vi "Window-Calibration toolbox.vi"() -> ()   [LabVIEW 2017]
uses:
  Configuration code/Calibration/ToolBox/TypeDefs/Current Calibration Parameters.ctl
  Configuration code/Calibration/ToolBox/TypeDefs/ProcedureState.ctl
  Typedefs/Objective selector control enum.ctl
  <vilib>/Math Plots/3D Math Plots/3D Surface/3D Surface XCtrl/3D Surface.xctl
  <vilib>/vision/Image Controls.llb/IMAQ Image.ctl
  Configuration code/Calibration/ToolBox/TypeDefs/Procedure_State.ctl
  Configuration code/Calibration/ToolBox/TypeDefs/Control Plane.ctl
  Typedefs/HW config states enum.ctl
  Peripherals Control/XYZ Stage/Typedefs/XYZ stage data.ctl
  Peripherals Control/XYZ Stage/Typedefs/XYZ stage states.ctl
  Peripherals Control/XYZ Stage/Typedefs/XYZ channel ring.ctl
  Global Variables/General Globals.vi
  Configuration code/Calibration/Globals/gl_Calibration globals.vi
  Global Variables/gl_UI Ctrl Refs.vi
  <vilib>/Math Plots/3D Math Plots/3D Surface/3D Surface Datatype/Public/Plot Helper (Matrix).vi
  <resource>/objmgr/IMAQImage.rc
  <vilib>/GPower/Array/GPArray.lvlib
  Global Variables/gl_Queues.vi
  <vilib>/Math Plots/3D Math Plots/3D Surface/3D Surface Datatype/3D Surface Datatype.lvclass
  <vilib>/GPower/Array/Library/Create/Random/CreateRandomI8.vi
panel:
  out "Focal Plane":sgl format="Z:%#_g"
  in  "Set focal plane":bool
  out "Z plane exec time":u32
  out "Stage XYZ Position":cluster{"X":sgl, "Y":sgl, "Z":sgl}
  out "3D Surface":refnum<class "3D Plot Datatype.lvclass">[](xcontrol)
  out "Intensity Graph":i16[][](graph)
  out "Image Pixels (I16)":i16[][](array[numeric])
  out "Stage Zeroed ? 2":bool
  out "AOL Z values":i32[](array[numeric])
  out "Motor Z values":i32[](array[numeric])
  out "mini steps":dbl=100.0
  out "LL":dbl=100.0 format="%#_g µm"
  out "UL":dbl=100.0 format="%#_g µm"
  in  "miniStep size":dbl=100.0 format="%#_g µm"
  in  "Sequence":bool
  out "Stage Zeroed ?":bool
  out "Z":sgl format="Z:%#_g"
  out "Y":sgl format="Y:%#_g"
  out "X":sgl format="X:%#_g"
  out "Progress":u8(slide) scale=0.0..21.0
  in  "Step Size":dbl=100.0 format="%#_g µm"
  in  "Natural Plane":bool
  in  "Move Down":bool
  in  "Move Up":bool
  in  "Current Objective":T1="Olympus  20X"
  out "error out":errorcluster
  out "Procedure":T2
  in  "Auto Focus":bool
  in  "Signal Channel":enum16{"Red", "Green"}(ring)
  in  "Message_FrontPanel":string
  in  "Cancel":bool
  in  "Abort":bool
  in  "Next":bool
  in  "N":i32=512
  in  "Reload":bool
  out "Stop_Ind":bool
  in  "Save config.ini":bool
  in  "Exit":bool
  in  "Calibration Tab":T3(tab)
  in  "Live Image intensity":cluster{i16, i16}(slide)={0, 2048} scale=0.0..4095.0
  in  "Visible(Grid)":bool
  in  "Grid Lines":u32=2 min=2 max=10 step=1
  out "Image":T4(plugin-control)
  out "Array":T4[](array[plugin-control])
  out "Analysis Graph":cluster{"X":dbl, "Y":dbl}[](graph)
  out "PSF Plot":cluster{"X":dbl, "Y":dbl}[](graph)
  out "PSF Image":T4(plugin-control)
  in  "Objectives":string(tree)
  out "Calibration.ini Path":path
  out "Calibration.ini":string
  in  "Step details":string
  in  "Step No":T5(ring)
  in  "Pockels Cell Value for pointing mode":dbl
  in  "auto-set pockel":bool
  in  "Calibration_min":dbl
  in  "Calibration_max":dbl
  in  "Search_min":dbl
  in  "Search_max":dbl
  in  "Testing Range (Norm)_max":dbl=1.0
  in  "Testing Range (Norm)_min":dbl=-1.0
  in  "Auto Calibration":bool
  in  "Measure PSF":bool
  in  "Calibration test type":T6(ring)
  in  "Test":bool
  in  "Calibrate":bool
  in  "Calibration type":T7(ring)
  in  "Current Calibration Parameters":T8
  # "Current XYZ Stage Position"
  # "Natural Focal Plane Z motor position must be \nset  to Zero before using the following buttons"
  # "Calibration Options"
  # "Maximal Search Range"
  # "to"
  # "(for sums &\ndiffs only)"
  # "Calibration Range from"
  # "to"
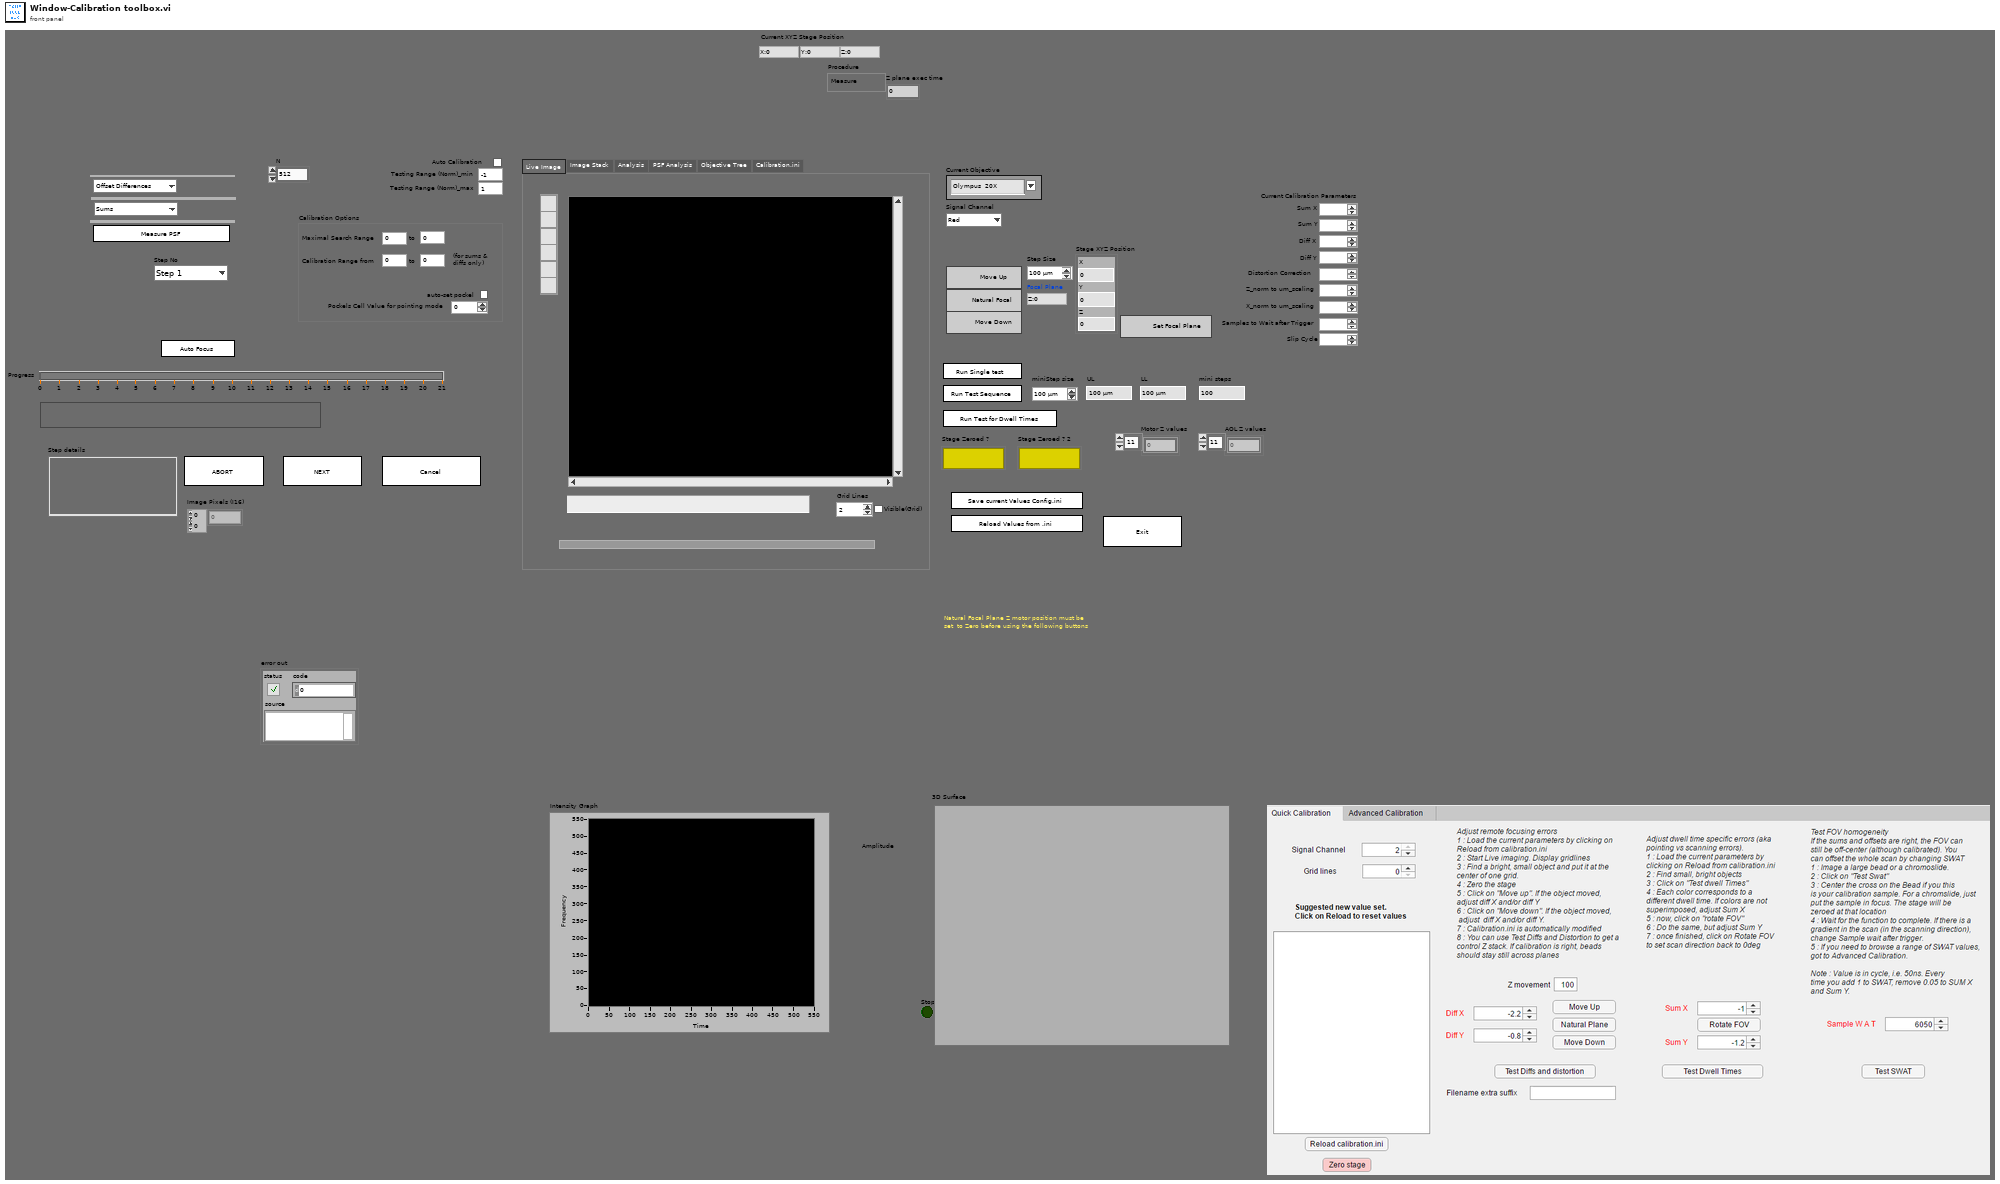
[diagram p1: front panel]
types:
  T1 = typedef "Objective selector control enum.ctl" = string
  T2 = typedef "ProcedureState.ctl" = enum16{"Measure", "Calibrate", "Sequence", "Test"}
  T3 = enum32{"Live Image", "Image Stack", "Analysis", "PSF Analysis", "Objective Tree", "Calibration.ini"}
  T4 = typedef "IMAQ Image.ctl" = refnum<image>
  T5 = enum16{"Step 1", "Step 2", "Step 3", "Step 4", "Step 5", "Step 6", "Step 7", "Step 8", "Step 9"}
  T6 = enum16{"Sums", "Diffs and Distortion", "Dwell Times"}
  T7 = enum16{"Offset Differences", "Magnification", "Offset Sums", "X-Y Scaling", "Z-Scaling"}
  T8 = typedef "Current Calibration Parameters.ctl" = cluster{"Sum X":dbl, "Sum Y":dbl, "Diff X":dbl, "Diff Y":dbl, "Distortion Correction":dbl, "Z_norm to um_scaling":dbl, "X_norm to um_scaling":dbl, "Samples to Wait after Trigger":dbl, "Slip Cycle":dbl}
  T9 = enum32{"Invalid", "Standard", "Closed", "Hidden", "Minimized", "Maximized"}
  T10 = typedef "HW config states enum.ctl" = enum16{"Load from file", "Save to file", "Write all", "Read all", "Write XY stage settings", "Write DAQ FPGA settings", "Write Control FPGA settings", "Write Phys Channels", "Write System Config", "Write HW Config", "Save System Config", "Save HW Config", "Clear", "Compare from file"}
  T11 = enum8{"Enabled", "Disabled", "Disabled and Grayed Out"}
  T12 = enum16{"Initialise", "Load from file", "Save to file", "Read", "Write"}
  T13 = enum32{"Bad", "Idle", "Run top level", "Running"}
  T14 = typedef "Live graph data queue ref.ctl" = refnum<queue>
  T15 = enum32{"Image", "Image Stack", "Analysis", "PSF Analysis", "Objective Tree", "Calibration.ini"}
  T16 = typedef "Calibration config.ctl" = cluster{"Current Objective":string, "Objective Settings":T17[], "PreChirper Values Preset ?":bool, "PreChirper Settings":T18[], "PreChirper Constants":T19}
  T17 = typedef "Objective Config.ctl" = cluster{"Name":string, "Sum X":dbl, "Sum Y":dbl, "Diff X":dbl, "Diff Y":dbl, "Distortion Correction":dbl, "Z_norm to um_scaling":dbl, "X_norm to um_scaling":dbl, "Calibrated Wavelength":dbl}
  T18 = typedef "Prechirper Cal Config.ctl" = cluster{"Wavelength":i32, "Prism 1":i32, "Prism 2":i32}
  T19 = typedef "PreChirper constants.ctl" = cluster{"a 1":i32, "b 1":i32, "c 1":i32, "a 2":i32, "b 2":i32, "c 2":i32, "lmin":i32, "lmax":i32}
  T20 = typedef "System Configuration.ctl" = cluster{"Laser wavelength (nm)":dbl, "DAQ FPGA System":T21, "Control system":T22}
  T21 = typedef "DAQ FPGA system config.ctl" = cluster{"Clock Freq (MHz) ":dbl, "Samples Wait after Trigger":u16, "AOD fill":u16, "StartupDelay":i32, "Slip Cycle (clock cycles)":u32, "Add Cycle":bool}
  T22 = typedef "CTRL system config.ctl" = cluster{"AOD 1 Amplitude":i16, "AOD 2 Amplitude":i16, "AOD 3 Amplitude":i16, "AOD 4 Amplitude":i16, "AOD 5 Amplitude":i16, "AOD 6 Amplitude":i16, "T0 (ns)":dbl, "Ta (ns)":dbl, "Data Time Interval (ns)":dbl, "Ctrl FPGA Clock (MHz)":dbl}
  T23 = typedef "UI ctrl refs cluster.ctl" = cluster{"Top level VI path":path, "Top level VI ref":refnum<vi>, "User menu ref":refnum<k9>, "Sub Panel control":refnum<vi>, "Imaging Param Tab":refnum<vi>, "Occurrence-Start drivers":refnum<k4>, "Occurrence-Speed logging initialised":refnum<k4>, "Occurrence-XYZ stage initialised":refnum<k4>, "Exit button":refnum<vi>, "Status ind":refnum<vi>, "Set as origin":refnum<vi>, "Speed Logging":refnum<vi>, "Time Lapse":refnum<vi>, "Live Imaging":refnum<vi>, "AOL Z Stack":refnum<vi>, "Motor Z Stack":refnum<vi>, "Funct Acq button":refnum<vi>, "Hard Shutter":refnum<vi>, "Virtual Shutter":refnum<vi>, "Laser Power":refnum<vi>, "AOL Mode":refnum<vi>, "Frame Size":refnum<vi>, "Field of View":refnum<vi>, "Dwell Time":refnum<vi>, "Zoom":refnum<vi>, "AOL Z":refnum<vi>, "Objective":refnum<vi>, "Axis":refnum<vi>, "Paths & Names":refnum<vi>, "Experiment folder path (ind.)":refnum<vi>, "Last State (Ind.)":refnum<vi>, "Averages":refnum<vi>, "Angle (degrees)":refnum<vi>, "X centre":refnum<vi>, "Y centre":refnum<vi>, "Plane Mode":refnum<vi>, "# Planes":refnum<vi>, "Z Start":refnum<vi>, "Z Stop":refnum<vi>, "Z Step":refnum<vi>, "PMT 1":refnum<vi>, "PMT 2":refnum<vi>, "Stage XYZ Position":refnum<vi>, "Pockels@Z Start":refnum<vi>, "Pockels@Z Stop":refnum<vi>, "Obtain Z Start":refnum<vi>, "Obtain Z Stop":refnum<vi>, "Live stim.trig.period":refnum<vi>, "Live stim.trig.enable":refnum<vi>, "Movement Correction":refnum<vi>, "Load Reference Image":refnum<vi>, "XY Stage Move":refnum<vi>, "MovCor Cluster":refnum<vi>, "RefDAQParam":refnum<vi>, "Funct. Acq. Pockels Modulation":refnum<vi>, "Ref Laser Power":refnum<vi>, "Enable Video Recording":refnum<vi>, "Video Record-Live Imaging":refnum<vi>, "Video Record-Funct acq":refnum<vi>, "Reference Source":refnum<vi>, "AOL Z-stack Chirps Ready (ind)":refnum<vi>, "Target time between mov.cor. ref triggers (ms)":refnum<vi>, "Funct. Acq. Ref frame save":refnum<vi>, "Tracking button":refnum<vi>, "Show ref plots window":refnum<vi>, "Center freq ind (nm)":refnum<vi>, "Pickup mode (ind)":refnum<vi>, "Logging queue (ind)":refnum<vi>, "Back aperture power (ind.)":refnum<vi>, "Power after objective (ind.)":refnum<vi>, "Switch user":refnum<vi>, "Ls1 Conn. Status":refnum<vi>, "Ls1Tuning Status":refnum<vi>, "Ls1 Faults":refnum<vi>, "Ls1 Connection":refnum<vi>, "Ls1 Mode":refnum<vi>, "Ls1 POWER [mW]":refnum<vi>, "Ls1Shutter":refnum<vi>, "Ls1 Wavelength":refnum<vi>, "Ls1 Note":refnum<vi>, "Ls1 Confirm Wav":refnum<vi>, "Ls1 PreChrp Prism1":refnum<vi>, "Ls1 PreChrp Prism2":refnum<vi>, "Ls1 wav top Ind":refnum<vi>, "Ls1 power top Ind":refnum<vi>, "Ls1 Pump peak Hold":refnum<vi>, "Ls1 Status Ind":refnum<vi>, "Ls1 wav cancel":refnum<vi>, "Experiment Type":refnum<vi>, "Biology Information":refnum<vi>}
  T24 = typedef "AOL Z cal process refs.ctl" = cluster{"This VI":refnum<vi>, "Abort (ind)":refnum<vi>, "Next (ind)":refnum<vi>, "Cancel":refnum<vi>, "Next":refnum<vi>, "Message":refnum<vi>, "Progress":refnum<vi>}
  T25 = typedef "Image Type" = u32
  T26 = typedef "Control Plane.ctl" = enum16{"XY-X", "XY-Y", "Z"}
  T27 = typedef "Procedure_State.ctl" = cluster{"Procedure":T2, "Parameter":T26, "Symmetric":bool}
  T28 = typedef "XYZ stage states.ctl" = enum16{"Dequeue", "Initialize", "Read Position", "Read Speed Setting", "Move", "Set Max Speed", "Reset Axis", "Stop all movement"}
  T29 = typedef "XYZ channel ring.ctl" = string
  T30 = typedef "XYZ stage data.ctl" = cluster{"Command":T28, "Channel":T29, "X":sgl, "Y":sgl, "Z":sgl, "Speed":i32, "Zero":bool, "Use acknowledgement?":bool}
  T31 = typedef "AOL_Globals.ctl" = cluster{"Imaging Protocol":T32, "Number of POI":u16, "Number of Miniscans":u16, "Number of Trials":u16, "Number of Cycles ":u64, "# Averaged Frames":u16, "Laser power (%)":u8, "Pockels (V)":dbl, "Acquisition Length (sec)":dbl, "Fill time (us)":dbl, "POI Dwell time (us)":dbl, "Miniscan Dwell time per pixel (us)":dbl, "PMT 1":dbl, "PMT 2":dbl, "Back Apperture (mA)":dbl, "Frame Size":T33, "Center Frequency":dbl, "Field of View (norm)":dbl, "DwellTime (us)":dbl, "Wavelength (nm)":dbl, "Zoom":dbl, "AOL Z":dbl, "AOL Mode":T34, "GridXY":dbl, "GridZ":dbl, "TriggerPeriod (sec)":dbl, "Number of Pixels in Miniscan":u16, "Experiment folder path":path, "X centre":dbl, "Y centre":dbl, "Angle (degrees)":dbl, "Plane Mode":T35, "Threshold":u16[], "Regenerate Chirps":bool, "Rectangle ROI length (pixels)":u16, "Rectangle ROI height (pixels)":u16, "AOD fill":u16, "StartupDelay":i32, "Samples Wait after Trigger":u16, "Slip Cycle":u32, "Add Cycle":bool, "Functional Mode":T36, "Z Start":dbl, "Z Stop":dbl, "# Planes":i32}
  T32 = typedef "Imaging Protocols enum.ctl" = enum16{"AOL Z-Stack", "Motor Z Stack", "Functional Acquisition", "Single Plane Acquisition", "Volume Acquisition", "Live Imaging", "Live Plane Imaging", "Live Volume Imaging"}
  T33 = typedef "Frame Size.ctl" = u16
  T34 = typedef "AOL modes.ctl" = enum16{"Raster", "Structural", "Pointing", "Mini Scan", "Alignment"}
  T35 = typedef "Plane Mode.ctl" = u16
  T36 = typedef "Functional Mode.ctl" = enum16{"Point", "Line", "Patch", "Plane", "Volume"}
  T37 = typedef "Live imaging queue element.ctl" = cluster{"Red channel":T4, "Green channel":T4, "Ref Red channel":T4, "Ref Green channel":T4, "Mov cor":bool}
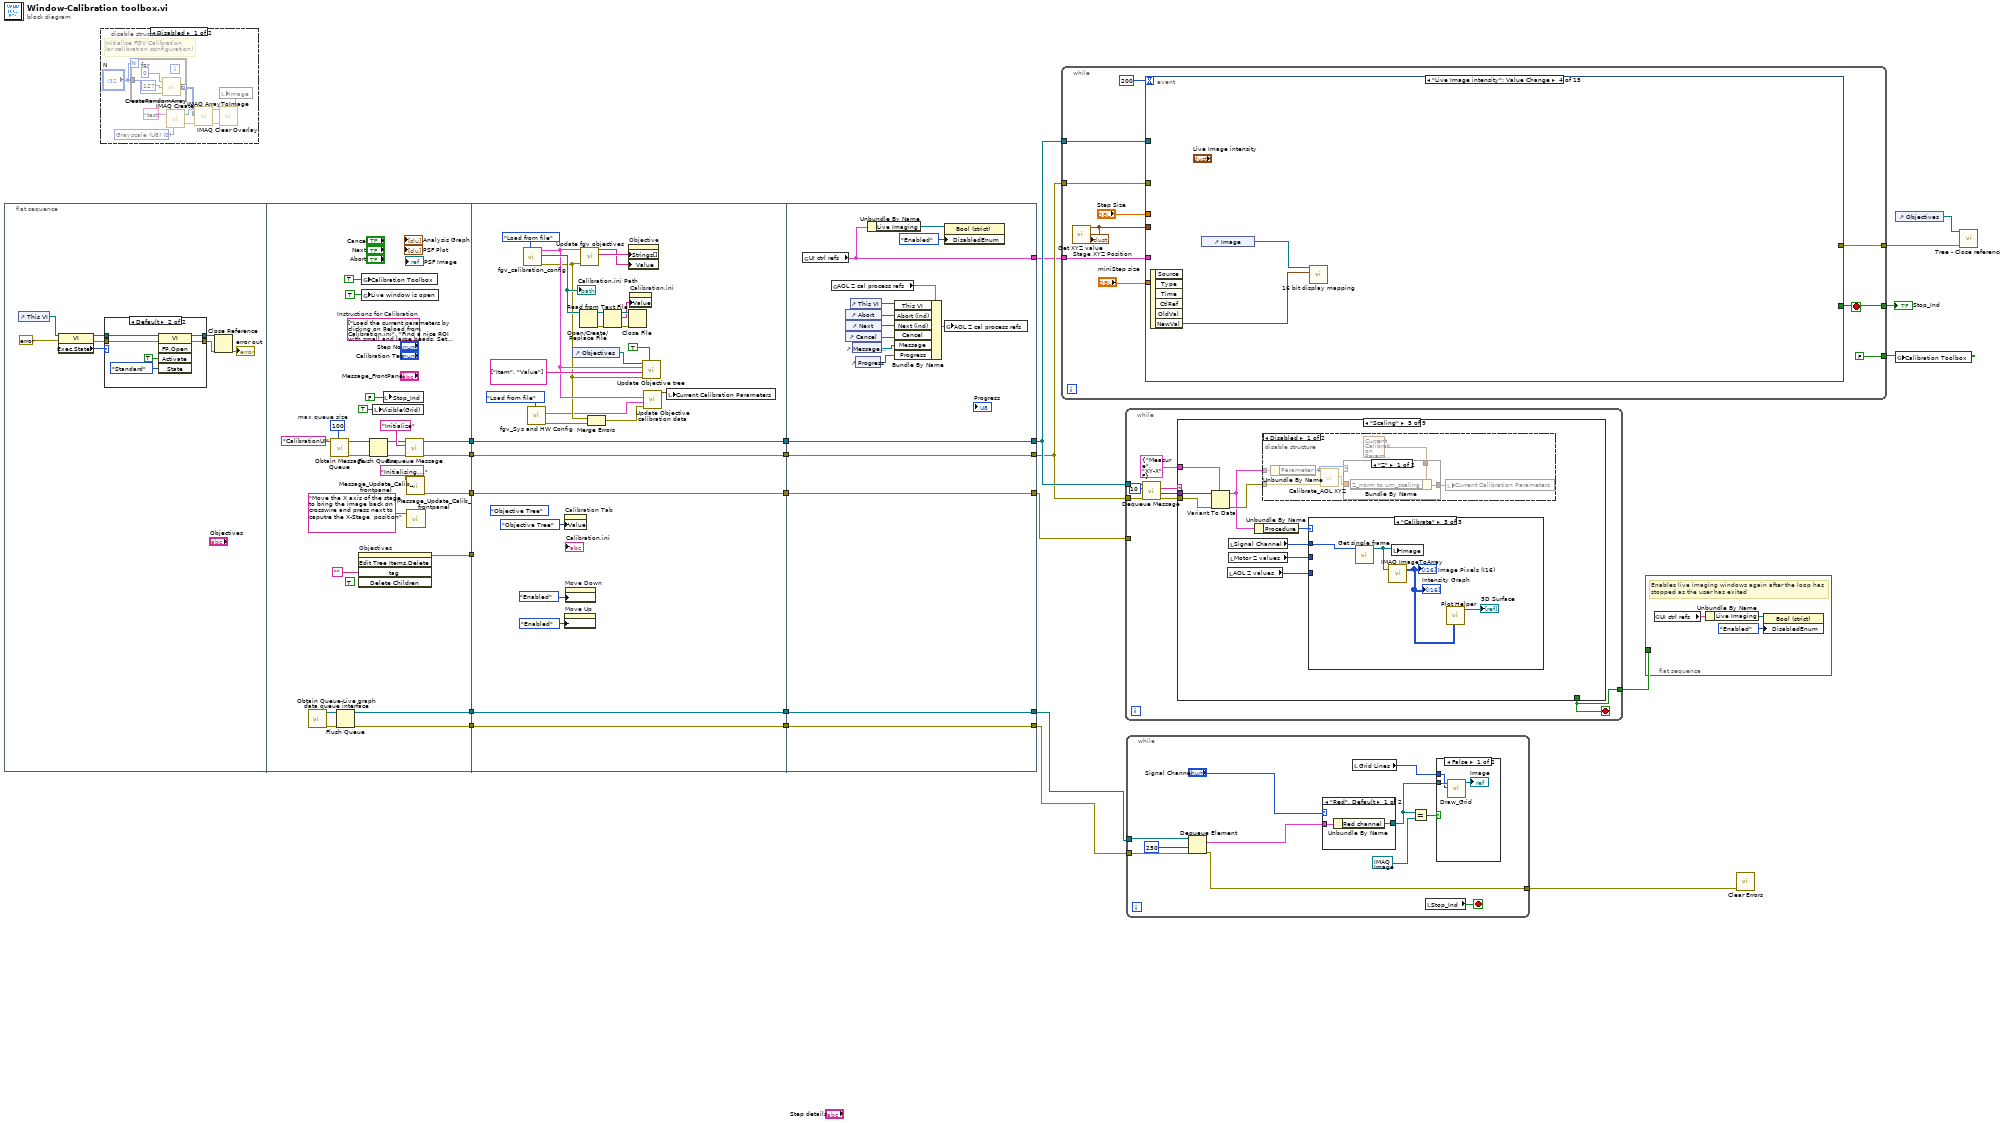
[diagram p0: block diagram]
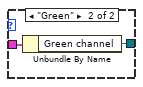
[diagram p3: hidden frame]
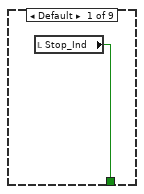
[diagram p6: hidden frame]
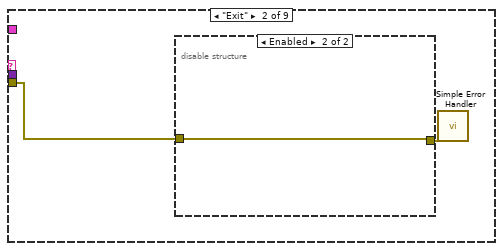
[diagram p7: hidden frame]
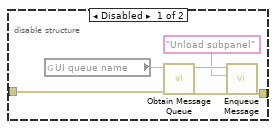
[diagram p8: hidden frame]
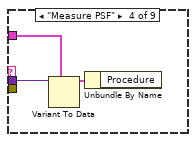
[diagram p10: hidden frame]
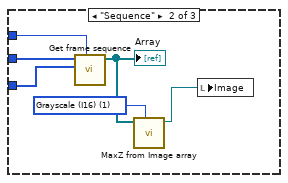
[diagram p12: hidden frame]
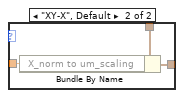
[diagram p13: hidden frame]
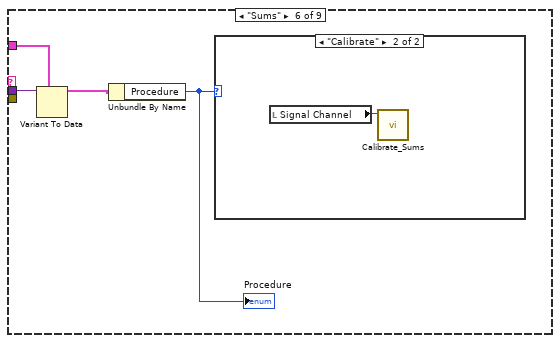
[diagram p15: hidden frame]
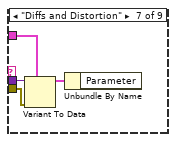
[diagram p17: hidden frame]
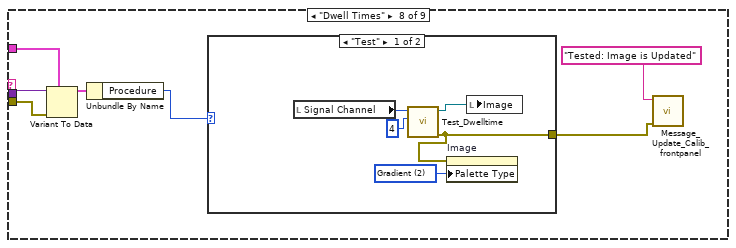
[diagram p18: hidden frame]
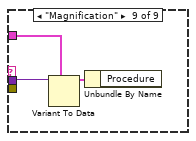
[diagram p20: hidden frame]
diagram:
  n1 = flat-sequence {
    tunnel: [w54] -> w15
    tunnel: [w53] -> w13
    tunnel: [w51] -> w11
    tunnel: [w44] -> w9
    tunnel: [w42] -> w7
    tunnel: [w41] -> w3
    tunnel: w15 -> [w88]
    tunnel: [w88] -> w14
    tunnel: w13 -> [w87]
    tunnel: [w87] -> w12
    tunnel: w11 -> [w86]
    tunnel: [w86] -> w10
    tunnel: w9 -> [w85]
    tunnel: [w85] -> w8
    tunnel: w7 -> [w84]
    tunnel: [w84] -> w6
    tunnel: w3 -> [_]
    tunnel: [w100] -> w17
    tunnel: [w101] -> w18
    tunnel: [w102] -> w19
    tunnel: [w103] -> w21
    tunnel: [w104] -> w22
    tunnel: w14 -> [w104]
    tunnel: w12 -> [w103]
    tunnel: w10 -> [w102]
    tunnel: w8 -> [w101]
    tunnel: w6 -> [w100]
    tunnel: [w92] -> w5
    frame #0 {
      n2 = control-ref of="This VI"() -> (w28:refnum<vi>)
      n3 = property class="VI"(reference=w28, error in=errorcluster {"status"=FALSE, "code"=0, "source"=""} ("error in (no error)")) -> (reference out=w27:refnum<vi>, error out=w26:errorcluster, "Exec.State"=w24:T13)
      n4 = case shown="Default" w24 {
        tunnel: [w33 w34] -> w31
        tunnel: [w32 w39] -> w30
        tunnel: w27 -> [w33 w36]
        tunnel: w26 -> [w32 w35]
        frame "Run top level" {
        }
        frame Default {
          n5 = invoke class="VI" method="FP.Open"(reference=w36, error in=w35, "Activate"=TRUE ("Activate?"), "State"=T9."Standard") -> (reference out=w34:refnum<vi>, error out=w39:errorcluster)  [unwired: 1 in, 3 out]
        }
      }
      n6 = Close Reference(reference=w31, error in (no error)=w30) -> (error out=→"error out":errorcluster)
    }
    frame #1 {
      (unwired) TRUE ("Delete Children?")
      w56 = 100  # max queue size
      (unwired) string[] ["Load the current parameters by clicking on Reload from Calibration.ini", "Find a nice ROI with small and large beads. Set PMT at 500 and adjust pockels", "Test FOV gives a sharp, single peak with Auto Focus. If yes, zero the stage. Otherwise change ROI", "Use 'Test Diffs and distortion' AND ' Test Sum' to see if the rig needs calibration for differences or sums.", "Process to teh necessary calibrations. If the performances are suboptimal, change ROI or incease laser", "If the results are bad, you can restore the previous settings by clicking on Reload from calibration.ini", "If calibration fails repetitively, try another magnification, laser pwer or FOV size.", "If calibration crashes in mid-process, go to Acquisition tab, reset drives and set the stage back to [0,0,0]. If you were in pointing mode, set teh mode toggie back to raster. Then check the pockels values."]  # Instructions for Calibration
      n7 = call "Obtain Queue-Live graph data queue interface.vi"() -> ("error out"=w45:errorcluster, "Live graphs queue"=w46:T14)  [unwired: 10 in]
      n8 = call "Obtain Message Queue.vi"("max queue size (-1, unlimited)"=w56, "Queue name"="CalibrationUI") -> ("error out"=w58:errorcluster, "Message Queue"=w60:refnum<queue>)  [unwired: 8 in]
      n9 = Flush Queue(queue=w46, error in (no error)=w45) -> (queue out=w44:T14, error out=w42:errorcluster)  [unwired: 1 out]
      n10 = invoke on="Objectives" class="Tree (strict)" method="Edit Tree Items.Delete"("tag"="") -> (error out=w41:errorcluster)  [unwired: 4 in, 4 out]
      n11 = global write "General Globals.vi" "Calibration Toolbox"(TRUE ("Calibration Toolbox")) -> ()
      n12 = global write "General Globals.vi" "Live window is open"(TRUE ("Live window is open")) -> ()
      n13 = Flush Queue(queue=w60, error in (no error)=w58) -> (queue out=w59:refnum<queue>, error out=w57:errorcluster)  [unwired: 1 out]
      n14 = local write "Visible(Grid)"(TRUE ("Visible(Grid)")) -> ()
      n15 = local write "Stop_Ind"(FALSE ("Stop_Ind")) -> ()
      n16 = call "Enqueue Message.vi"("error in (no error)"=w57, "Message"="Initialize", "Queue"=w59) -> ("error out"=w53:errorcluster, "Queue out"=w54:refnum<queue>)  [unwired: 7 in]
      n17 = call "Message_Update_Calib_frontpanel.vi"("Message"="Initialising....") -> ("error out"=w51:errorcluster)  [unwired: 10 in]
      n18 = call "Message_Update_Calib_frontpanel.vi"("Message"="Move the X axis of the stage to bring the image back on crosswire and press next to caputre the X-Stage  position") -> ()  [unwired: 10 in, 1 out]
    }
    frame #2 {
      (unwired) T15."Objective Tree" ("Calibration Tab")
      n19 = call "fgv_calibration_config.vi"("Cal config ops"=T12."Load from file") -> ("error out"=w66:errorcluster, "File Path"=w72:path, "Config cluster OUT"=w70:T16)  [unwired: 8 in]
      "Calibration.ini Path" <- w72
      n20 = call "fgv_Sys and HW Config.vi"("Function"=HW_config_states_enum."Load from file") -> ("error out"=w65:errorcluster, "System Config OUT"=w63:T20)  [unwired: 8 in, 1 out]
      n21 = property on="Calibration Tab" class="TabCtl (strict)"("Value"=T3."Objective Tree" ("Calibration Tab")) -> ()  [unwired: 2 in, 2 out]
      n22 = property on="Move Up" class="Bool"("DisabledEnum"=T11."Enabled" ("Disabled")) -> ()  [unwired: 2 in, 2 out]
      n23 = property on="Move Down" class="Bool"("DisabledEnum"=T11."Enabled" ("Disabled")) -> ()  [unwired: 2 in, 2 out]
      n24 = control-ref of="Objectives"() -> (w75:refnum<vi>)
      n25 = Open/Create/Replace File(file path (use dialog)=w72) -> (refnum out=w80:refnum<file>, error out=w79:errorcluster)  [unwired: 5 in, 1 out]
      n26 = call "Update fgv objectives.vi"("error in (no error)"=w66, "Config cluster IN"=w70) -> ("Available Objectives"=w77:string[], "Current Objective"=w76:string)  [unwired: 7 in, 1 out]
      n27 = Merge Errors(w66, w65) -> (w64:errorcluster)
      n28 = Read from Text File(file (use dialog)=w80, error in=w79) -> (refnum out=w81:refnum<file>, text=w78:string, error out=w82:errorcluster)  [unwired: 2 in, 1 out]
      n29 = property on="Objective" class="CmbBox (strict)"("Strings[]"=w77, "Value"=w76) -> ()  [unwired: 2 in, 2 out]
      n30 = Close File(refnum=w81, error in=w82) -> ()  [unwired: 2 out]
      n31 = property on="Calibration.ini" class="Str"("Value"=w78) -> ()  [unwired: 2 in, 2 out]
      n32 = call "Update Objective tree.vi"("Visible Items:Column Headers Visible"=TRUE, "error in (no error)"=w66, "Column Header Strings[]"=string[] ["Item", "Value"], "Config cluster IN"=w70, "TreeControl in"=w75) -> ()  [unwired: 6 in, 1 out]
      n33 = call "Update Objective calibration data.vi"("error in (no error)"=w64, "System Config"=w63, "Config cluster OUT"=w70) -> ("Current Calibration Parameters out"=w71:T8)  [unwired: 7 in, 1 out]
      n34 = local write "Current Calibration Parameters"(w71) -> ()
    }
    frame #3 {
      n35 = global read "gl_UI Ctrl Refs.vi" "UI ctrl refs"() -> (w92:T23)
      n36 = global read "gl_Calibration globals.vi" "AOL Z cal process refs"() -> (w94:T24)
      n37 = control-ref of="Abort"() -> (w93:refnum<vi>)
      n38 = control-ref of="Next"() -> (w99:refnum<vi>)
      n39 = control-ref of="Cancel"() -> (w95:refnum<vi>)
      n40 = control-ref of="This VI"() -> (w98:refnum<vi>)
      n41 = control-ref of="Message_FrontPanel"() -> (w96:refnum<vi>)
      n42 = control-ref of="Progress"() -> (w89:refnum<vi>)
      n43 = Unbundle By Name(w92) -> ("Live Imaging"=w91:refnum<vi>)
      n44 = Bundle By Name(cluster=w94, "This VI"=w98, "Abort (ind)"=w93, "Next (ind)"=w99, "Cancel"=w95, "Message"=w96, "Progress"=w89) -> (w97:T24)
      n45 = property class="Bool (strict)"(reference=w91, "DisabledEnum"=T11."Enabled" ("Disabled")) -> ()  [unwired: 1 in, 2 out]
      n46 = global write "gl_Calibration globals.vi" "AOL Z cal process refs"(w97) -> ()
    }
  }
  n47 = disable-structure shown="Disabled" {
    frame Disabled {
      w112 = T25 0 items=["Grayscale (U8)", "Grayscale (I16)", "Grayscale (SGL)", "Complex (CSG)", "RGB (U32)", "HSL (U32)", "RGB (U64)", "Grayscale (U16)"] ("Image Type")
      # "Initialise FGV Calibration\n(or calibration configuration)"
      n48 = for {
        N: "N" -> [_]
        tunnel: [w115] -> w109 mode=indexing
        tunnel: "N" -> [w114]
        n49 = call-poly <vilib>:"CreateRandomArray.vi"("N"=w114, "Maximum value"=i8 127, "Minimum value"=i8 0) -> ("Created array"=w115:i8[])
      }
      n50 = call "IMAQ Create"("Image Name"="test", "Image Type"=w112) -> ("New Image"=w110:T4, "error out"=w111:errorcluster)  [unwired: 3 in]
      n51 = call "IMAQ ArrayToImage"("error in (no error)"=w111, "Image Pixels (U8)"=w109, "Image"=w110) -> ("error out"=w106:errorcluster, "Image Out"=w107:T4)  [unwired: 7 in]
      n52 = call "IMAQ Clear Overlay"("error in (no error)"=w106, "Image"=w107) -> ("Image Out"=w105:T4)  [unwired: 8 in, 1 out]
      n53 = local write "Image"(w105) -> ()
    }
    frame Enabled {
    }
  }
  n54 = while {
    tunnel: [w127] -> w23
    tunnel: w22 -> [w126]
    tunnel: w21 -> [w123]
    tunnel: [FALSE ("Calibration Toolbox")] -> w20
    tunnel: w5 -> [w122]
    tunnel: [w121] -> w2
    stop <- w127 stop-if-true
    n55 = call "Get XYZ value.vi"() -> ("Stage XYZ Position"=w118:cluster{"X":sgl, "Y":sgl, "Z":sgl})  [unwired: 11 in]
    "Stage XYZ Position" <- w118
    n56 = event shown="[3] \"Live Image intensity\": Value Change" {
      selector: _ -> [_ _ _ _ _ _ _ _ _ _ _ _ _ _ _]
      dyn-events: _ -> [_ _ _ _ _ _ _ _ _ _ _ _ _ _ _]
      timeout: 200 -> [_ _ _ _ _ _ _ _ _ _ _ _ _ _ _]
      tunnel: [_ TRUE _ _ _ _ _ _ _ _ _ _ _ _ _] -> w127
      tunnel: w126 -> [_ w144 _ _ _ _ _ w252 w306 w358 _ w381 _ _ _]
      tunnel: w123 -> [_ _ _ _ _ _ _ _ _ _ _ _ _ _ _]
      tunnel: w122 -> [_ _ _ _ w172 _ _ w250 w305 w348 _ _ _ _ _]
      tunnel: [_ _ _ _ _ _ _ _ _ _ _ _ w387 _ _] -> w121
      tunnel: "Step Size" -> [w131 _ _ _ w160 w239 _ _ _ _ _ _ _ _ _]
      tunnel: "miniStep size" -> [w130 _ _ _ _ w235 _ _ _ _ _ _ _ _ _]
      tunnel: w118 -> [w129 _ w153 _ w159 _ _ _ _ _ _ _ _ _ _]
      event Timeout {
        n57 = event-data() -> ()  [unwired: 1 in, 3 out]
        n58 = First Call?() -> (First Call?: T/F=w132:bool)
        n59 = Unbundle By Name(w129) -> ("X"=→"X":sgl, "Y"=→"Y":sgl, "Z"=w128:sgl)
        "Z" <- w128
        n60 = case shown="True" w132 {
          tunnel: w131 -> [_ w142]
          tunnel: w130 -> [_ w141]
          tunnel: w128 -> [_ w135]
          frame False {
          }
          frame True {
            n61 = Absolute Value(x=w142) -> (abs(x)=w140:dbl)
            n62 = local write "Focal Plane"(w135) -> ()
            n63 = Negate(x=w140) -> (-x=w139:dbl)
            n64 = call "Calculate Z step size.vi"("Step"=w141, "Stop"=w139, "Start"=w140) -> ("AOL Z values"=w136:i32[], "Motor Z values"=w137:i32[], "Number of steps"=w138:i32)  [unwired: 6 in]
            n65 = local write "LL"(w139) -> ()
            n66 = local write "UL"(w140) -> ()
            n67 = local write "AOL Z values"(w136) -> ()
            n68 = local write "mini steps"(w138) -> ()
            n69 = local write "Motor Z values"(w137) -> ()
          }
        }
      }
      event Panel Close; "Exit": Value Change {
        n70 = event-data() -> ()  [unwired: 1 in, 2 out]
        n71 = case shown="True" "Exit" {
          tunnel: w144 -> [_ w151]
          frame False {
          }
          frame True {
            (unwired) enum16{"X-Y", "Z"}."X-Y" ("Parameter")
            n72 = Bundle By Name(cluster=T27 {"Procedure"=enum."Measure", "Parameter"=enum."XY-X", "Symmetric"=FALSE} ("input cluster"), "Procedure"=ProcedureState."Measure", "Parameter"=Control_Plane."XY-X") -> (w148:T27)
            n73 = call "Enqueue Message.vi"("Message Data"=w148, "Message"="Exit", "Queue"=w151) -> ()  [unwired: 7 in, 2 out]
          }
        }
      }
      event "Set focal plane": Value Change {
        n74 = event-data() -> ()  [unwired: 1 in, 6 out]
        n75 = Unbundle By Name(w153) -> ("Z"=→"Focal Plane":sgl)
      }
      event "Live Image intensity": Value Change {
        n76 = event-data() -> ("NewVal"=w155:cluster{i16, i16})  [unwired: 1 in, 5 out]
        n77 = control-ref of="Image"() -> (w154:refnum<vi>)
        n78 = call "16 bit display mapping.vi"("16 bit display mapping"=w155, "Image Display"=w154) -> ()  [unwired: 8 in, 2 out]
      }
      event "Move Up", "Move Down", "Natural Plane": Value Change {
        n79 = event-data() -> ("CtlRef"=w175:refnum<vi>)  [unwired: 1 in, 3 out]
        n80 = Unbundle By Name(w159) -> ("Z"=w158:sgl)
        n81 = Unbundle By Name(w172) -> ("AOL Z"=w171:refnum<vi>)
        n82 = property class="Bool"(reference=w175) -> (error out=w173:errorcluster, "Label.Text"=w174:string)  [unwired: 1 in, 1 out]
        n83 = flat-sequence {
          tunnel: w174 -> [w179]
          tunnel: w173 -> [w182]
          tunnel: [w181] -> w168
          tunnel: [w180] -> w166
          tunnel: [w179] -> w164
          tunnel: [w178] -> w161
          tunnel: w160 -> [w177]
          tunnel: w158 -> [w176]
          tunnel: w168 -> [w198]
          tunnel: [w198] -> w167
          tunnel: w166 -> [w197]
          tunnel: [w197] -> w165
          tunnel: w164 -> [w196]
          tunnel: [w196] -> w163
          tunnel: [w193] -> w162
          tunnel: w161 -> [w194]
          tunnel: [w192] -> w156
          tunnel: w167 -> [w207]
          tunnel: w165 -> [w206]
          tunnel: w171 -> [w205]
          tunnel: [w204] -> w170
          tunnel: w163 -> [w204]
          tunnel: w162 -> [w203]
          tunnel: [w203] -> w169
          tunnel: [w201] -> w157
          tunnel: w156 -> [w201]
          tunnel: w170 -> [w225]
          tunnel: w169 -> [w224]
          tunnel: w157 -> [w220]
          frame #0 {
            n84 = global read "gl_Calibration globals.vi" "AOL Z cal process refs"() -> (w178:T24)
            n85 = case shown="\"Natural Plane\", Default" w179 {
              tunnel: w182 -> [_ _ _]
              tunnel: w177 -> [_ w185 w190]
              tunnel: [0.0 ("Step Size") w188 w190] -> w180
              tunnel: [w183 w186 w189] -> w181
              tunnel: w176 -> [_ w187 w191]
              frame "Natural Plane", Default {
                n86 = local read "Focal Plane"() -> (w183:sgl)
              }
              frame "Move Up" {
                n87 = Add(x=w185, y=w187) -> (x+y=w186:dbl)
                n88 = Negate(x=w185) -> (-x=w188:dbl)
              }
              frame "Move Down" {
                n89 = Subtract(x=w191, y=w190) -> (x-y=w189:dbl)
              }
            }
          }
          frame #1 {
            n90 = Unbundle By Name(w194) -> ("Message"=w193:refnum<vi>)
            n91 = disable-structure shown="Disabled" {
              frame Disabled {
                w199 = T11."Disabled and Grayed Out" ("Disabled")
                n92 = property on="Move Up" class="Bool"("DisabledEnum"=w199) -> ()  [unwired: 2 in, 2 out]
                n93 = property on="Move Down" class="Bool"("DisabledEnum"=w199) -> ()  [unwired: 2 in, 2 out]
                n94 = property on="Natural Plane" class="Bool"("DisabledEnum"=w199) -> ()  [unwired: 2 in, 2 out]
              }
              frame Enabled {
              }
            }
            n95 = property class="Str"(reference=w193, "Value"="Adjusting...") -> ()  [unwired: 1 in, 2 out]
            n96 = Tick Count (ms)() -> (millisecond timer value=w192:u32)
          }
          frame #2 {
            n97 = disable-structure shown="Enabled" {
              disable-tunnel: [w217 errorcluster {"status"=FALSE, "code"=0, "source"=""} ("error in")] -> w211
              disable-tunnel: w206 -> [w216 _]
              disable-tunnel: w205 -> [w215 _]
              frame Disabled {
                n98 = property class="Slide (strict)"(reference=w215, "Value"=w216) -> (error out=w217:errorcluster)  [unwired: 1 in, 1 out]
                n99 = call "fgv_AOL_Globals Read.vi"() -> ("AOL_Globals"=w213:T31)  [unwired: 9 in, 2 out]
                n100 = Bundle By Name(cluster=w213, "AOL Z"=w216) -> (w214:T31)
                n101 = call "fgv_AOL_Globals Write.vi"("AOL_Globals"=w214) -> ()  [unwired: 10 in, 1 out]
              }
              frame Enabled {
              }
            }
            n102 = Bundle By Name(cluster=T30 {"Command"=enum."Initialize", "Channel"="Z", "X"=0.0, "Y"=0.0, "Z"=0.0, "Speed"=0, "Zero"=FALSE, "Use acknowledgement?"=TRUE} ("XYZ Stage data to queue"), "Command"=XYZ_stage_states."Move", "Channel"=T29 "Z", "Z"=w207, "Use acknowledgement?"=FALSE) -> (w212:T30)
            n103 = call "XYZ Stage-Command request module.vi"("error in"=w211, "Command"=XYZ_stage_states."Move", "XYZ Stage data to queue"=w212) -> ()  [unwired: 4 in, 5 out]
          }
          frame #3 {
            n104 = disable-structure shown="Disabled" {
              disable-tunnel: w225 -> [w226 _]
              frame Disabled {
                n105 = case shown="\"Natural Plane\", Default" w226 {
                  frame "Move Up" {
                    n106 = property on="Move Down" class="Bool"("DisabledEnum"=T11."Enabled" ("Disabled")) -> ()  [unwired: 2 in, 2 out]
                    n107 = property on="Move Up" class="Bool"("DisabledEnum"=T11."Disabled and Grayed Out" ("Disabled")) -> ()  [unwired: 2 in, 2 out]
                  }
                  frame "Move Down" {
                    n108 = property on="Move Up" class="Bool"("DisabledEnum"=T11."Enabled" ("Disabled")) -> ()  [unwired: 2 in, 2 out]
                    n109 = property on="Move Down" class="Bool"("DisabledEnum"=T11."Disabled and Grayed Out" ("Disabled")) -> ()  [unwired: 2 in, 2 out]
                  }
                  frame "Natural Plane", Default {
                    n110 = property on="Move Up" class="Bool"("DisabledEnum"=T11."Enabled" ("Disabled")) -> ()  [unwired: 2 in, 2 out]
                    n111 = property on="Move Down" class="Bool"("DisabledEnum"=T11."Enabled" ("Disabled")) -> ()  [unwired: 2 in, 2 out]
                  }
                }
              }
              frame Enabled {
              }
            }
            n112 = Tick Count (ms)() -> (millisecond timer value=w221:u32)
            n113 = Subtract(x=w221, y=w220) -> (x-y=→"Z plane exec time":u32)
            n114 = property on="Natural Plane" class="Bool"("DisabledEnum"=T11."Enabled" ("Disabled")) -> ()  [unwired: 2 in, 2 out]
            n115 = property class="Str"(reference=w224, "Value"="Done") -> ()  [unwired: 1 in, 2 out]
          }
        }
      }
      event "Step Size", "miniStep size": Value Change {
        n116 = event-data() -> ()  [unwired: 1 in, 6 out]
        n117 = Absolute Value(x=w239) -> (abs(x)=w238:dbl)
        "UL" <- w238
        n118 = Negate(x=w238) -> (-x=w237:dbl)
        "LL" <- w237
        n119 = call "Calculate Z step size.vi"("Step"=w235, "Stop"=w237, "Start"=w238) -> ("AOL Z values"=→"AOL Z values":i32[], "Motor Z values"=→"Motor Z values":i32[], "Number of steps"=→"mini steps":i32)  [unwired: 6 in]
      }
      event "Save config.ini": Value Change {
        n120 = event-data() -> ()  [unwired: 1 in, 6 out]
      }
      event "Calibrate": Value Change {
        (unwired) T15."Image" ("Calibration Tab")
        n121 = event-data() -> ("NewVal"=w253:bool)  [unwired: 1 in]
        n122 = Unbundle By Name(w250) -> ("Stage XYZ Position"=w249:refnum<vi>)
        n123 = property class="Clust (strict)"(reference=w249) -> ("Value"=w248:cluster{"X":sgl, "Y":sgl, "Z":sgl})  [unwired: 1 in, 2 out]
        n124 = Unbundle By Name(w248) -> ("X"=w247:sgl, "Y"=w246:sgl, "Z"=w245:sgl)
        n125 = Equal To 0?(x=w247) -> (x = 0?=w244:bool)
        n126 = Equal To 0?(x=w246) -> (x = 0?=w243:bool)
        n127 = Equal To 0?(x=w245) -> (x = 0?=w242:bool)
        n128 = Compound Arithmetic op=AND(w244, w243, w242) -> (w241:bool)
        n129 = case shown="True" w241 {
          selector: w241 -> [_ w254]
          frame False {
          }
          frame True {
            "Stage Zeroed ?" <- w254
          }
        }
        n130 = case shown="True" w253 {
          tunnel: w252 -> [_ w257]
          tunnel: "Calibration type" -> [_ w256]
          frame False {
          }
          frame True {
            n131 = case shown="True" TRUE {
              tunnel: w257 -> [_ w266]
              tunnel: w256 -> [_ w264]
              frame False {
                n132 = One Button Dialog(message="Please move the bead to a central position and\n'zero' the XYZ stage ") -> ()  [unwired: 1 in, 1 out]
              }
              frame True {
                (unwired) enum16{"X-Y", "Z"}."X-Y" ("Parameter")
                n133 = Bundle By Name(cluster=T27 {"Procedure"=enum."Measure", "Parameter"=enum."XY-X", "Symmetric"=FALSE} ("input cluster"), "Procedure"=ProcedureState."Calibrate", "Parameter"=Control_Plane."XY-X") -> (w260:T27)
                n134 = disable-structure shown="Enabled" {
                  disable-tunnel: [w270 w294] -> w267
                  disable-tunnel: [w269 w293] -> w265
                  disable-tunnel: w264 -> [w268 _]
                  disable-tunnel: "Scaling" ("Message") -> [_ w294]
                  disable-tunnel: w260 -> [_ w293]
                  frame Disabled {
                    n135 = case shown="\"Z-Scaling\"" w268 {
                      tunnel: ["Diffs and Distortion" ("Message") "Magnification" ("Message") "Sums" ("Message") "Scaling" ("Message") "Scaling" ("Message")] -> w270
                      tunnel: [w272 w277 w281 w286 w291] -> w269
                      frame "Offset Differences", Default {
                        n136 = Bundle By Name(cluster=T27 {"Procedure"=enum."Measure", "Parameter"=enum."XY-X", "Symmetric"=FALSE} ("input cluster"), "Procedure"=ProcedureState."Calibrate") -> (w272:T27)
                      }
                      frame "Magnification" {
                        n137 = Bundle By Name(cluster=T27 {"Procedure"=enum."Measure", "Parameter"=enum."XY-X", "Symmetric"=FALSE} ("input cluster"), "Procedure"=ProcedureState."Calibrate") -> (w277:T27)
                      }
                      frame "Offset Sums" {
                        n138 = Bundle By Name(cluster=T27 {"Procedure"=enum."Measure", "Parameter"=enum."XY-X", "Symmetric"=FALSE} ("input cluster"), "Procedure"=ProcedureState."Calibrate") -> (w281:T27)
                      }
                      frame "X-Y Scaling" {
                        n139 = Bundle By Name(cluster=T27 {"Procedure"=enum."Measure", "Parameter"=enum."XY-X", "Symmetric"=FALSE} ("input cluster"), "Procedure"=ProcedureState."Calibrate", "Parameter"=enum16{"X-Y", "Z"}."X-Y") -> (w286:T27)
                      }
                      frame "Z-Scaling" {
                        n140 = Bundle By Name(cluster=T27 {"Procedure"=enum."Measure", "Parameter"=enum."XY-X", "Symmetric"=FALSE} ("input cluster"), "Procedure"=ProcedureState."Calibrate", "Parameter"=enum16{"X-Y", "Z"}."Z") -> (w291:T27)
                      }
                    }
                  }
                  frame Enabled {
                  }
                }
                n141 = call "Enqueue Message.vi"("Message Data"=w265, "Message"=w267, "Queue"=w266) -> ()  [unwired: 7 in, 2 out]
              }
            }
          }
        }
        n142 = property on="Calibration Tab" class="TabCtl (strict)"("Value"=T3."Live Image" ("Calibration Tab")) -> ()  [unwired: 2 in, 2 out]
      }
      event "Sequence": Value Change {
        (unwired) T15."Image" ("Calibration Tab")
        n143 = event-data() -> ("NewVal"=w307:bool)  [unwired: 1 in]
        n144 = Unbundle By Name(w305) -> ("Stage XYZ Position"=w304:refnum<vi>)
        n145 = property class="Clust (strict)"(reference=w304) -> ("Value"=w303:cluster{"X":sgl, "Y":sgl, "Z":sgl})  [unwired: 1 in, 2 out]
        n146 = Unbundle By Name(w303) -> ("X"=w302:sgl, "Y"=w301:sgl, "Z"=w300:sgl)
        n147 = Equal To 0?(x=w302) -> (x = 0?=w299:bool)
        n148 = Equal To 0?(x=w301) -> (x = 0?=w298:bool)
        n149 = Equal To 0?(x=w300) -> (x = 0?=w297:bool)
        n150 = Compound Arithmetic op=AND(w299, w298, w297) -> (w296:bool)
        n151 = case shown="True" w296 {
          selector: w296 -> [_ w308]
          frame False {
          }
          frame True {
            "Stage Zeroed ? 2" <- w308
          }
        }
        n152 = case shown="True" w307 {
          tunnel: w306 -> [_ w310]
          frame False {
          }
          frame True {
            n153 = case shown="True" TRUE {
              tunnel: w310 -> [_ w318]
              frame False {
                n154 = One Button Dialog(message="Please move the bead to a central position and\n'zero' the XYZ stage ") -> ()  [unwired: 1 in, 1 out]
              }
              frame True {
                (unwired) enum16{"X-Y", "Z"}."X-Y" ("Parameter")
                n155 = Bundle By Name(cluster=T27 {"Procedure"=enum."Measure", "Parameter"=enum."XY-X", "Symmetric"=FALSE} ("input cluster"), "Procedure"=ProcedureState."Sequence", "Parameter"=Control_Plane."XY-X") -> (w313:T27)
                n156 = disable-structure shown="Enabled" {
                  disable-tunnel: [w322 w346] -> w319
                  disable-tunnel: [w321 w345] -> w317
                  disable-tunnel: _ -> [w320 _]
                  disable-tunnel: "Scaling" ("Message") -> [_ w346]
                  disable-tunnel: w313 -> [_ w345]
                  frame Disabled {
                    n157 = case shown="\"Z-Scaling\"" w320 {
                      tunnel: ["Diffs and Distortion" ("Message") "Magnification" ("Message") "Sums" ("Message") "Scaling" ("Message") "Scaling" ("Message")] -> w322
                      tunnel: [w324 w329 w333 w338 w343] -> w321
                      frame "Offset Differences", Default {
                        n158 = Bundle By Name(cluster=T27 {"Procedure"=enum."Measure", "Parameter"=enum."XY-X", "Symmetric"=FALSE} ("input cluster"), "Procedure"=ProcedureState."Calibrate") -> (w324:T27)
                      }
                      frame "Magnification" {
                        n159 = Bundle By Name(cluster=T27 {"Procedure"=enum."Measure", "Parameter"=enum."XY-X", "Symmetric"=FALSE} ("input cluster"), "Procedure"=ProcedureState."Calibrate") -> (w329:T27)
                      }
                      frame "Offset Sums" {
                        n160 = Bundle By Name(cluster=T27 {"Procedure"=enum."Measure", "Parameter"=enum."XY-X", "Symmetric"=FALSE} ("input cluster"), "Procedure"=ProcedureState."Calibrate") -> (w333:T27)
                      }
                      frame "X-Y Scaling" {
                        n161 = Bundle By Name(cluster=T27 {"Procedure"=enum."Measure", "Parameter"=enum."XY-X", "Symmetric"=FALSE} ("input cluster"), "Procedure"=ProcedureState."Calibrate", "Parameter"=enum16{"X-Y", "Z"}."X-Y") -> (w338:T27)
                      }
                      frame "Z-Scaling" {
                        n162 = Bundle By Name(cluster=T27 {"Procedure"=enum."Measure", "Parameter"=enum."XY-X", "Symmetric"=FALSE} ("input cluster"), "Procedure"=ProcedureState."Calibrate", "Parameter"=enum16{"X-Y", "Z"}."Z") -> (w343:T27)
                      }
                    }
                  }
                  frame Enabled {
                  }
                }
                n163 = call "Enqueue Message.vi"("Message Data"=w317, "Message"=w319, "Queue"=w318) -> ()  [unwired: 7 in, 2 out]
              }
            }
          }
        }
        n164 = property on="Calibration Tab" class="TabCtl (strict)"("Value"=T3."Live Image" ("Calibration Tab")) -> ()  [unwired: 2 in, 2 out]
      }
      event "Test": Value Change {
        n165 = event-data() -> ("NewVal"=w359:bool)  [unwired: 1 in]
        n166 = Unbundle By Name(w348) -> ("Stage XYZ Position"=w356:refnum<vi>)
        n167 = property class="Clust (strict)"(reference=w356) -> ("Value"=w355:cluster{"X":sgl, "Y":sgl, "Z":sgl})  [unwired: 1 in, 2 out]
        n168 = Unbundle By Name(w355) -> ("X"=w354:sgl, "Y"=w353:sgl, "Z"=w352:sgl)
        n169 = Equal To 0?(x=w354) -> (x = 0?=w351:bool)
        n170 = Equal To 0?(x=w353) -> (x = 0?=w350:bool)
        n171 = Equal To 0?(x=w352) -> (x = 0?=w349:bool)
        n172 = Compound Arithmetic op=OR(w351, w350, w349) -> (w347:bool)
        n173 = case shown="True" w359 {
          tunnel: w358 -> [_ w361]
          tunnel: "Calibration test type" -> [_ w362]
          tunnel: w347 -> [_ w360]
          frame False {
          }
          frame True {
            n174 = case shown="True" w360 {
              tunnel: w362 -> [_ w365]
              tunnel: w361 -> [_ w364]
              frame False {
                n175 = One Button Dialog(message="Please move the bead to a central position and\n'zero' the XYZ stage ") -> ()  [unwired: 1 in, 1 out]
              }
              frame True {
                n176 = case shown="\"Dwell Times\"" w365 {
                  tunnel: ["Sums" ("Message") "Diffs and Distortion" ("Message") "Dwell Times" ("Message")] -> w367
                  tunnel: [w369 w374 w378] -> w366
                  frame "Sums", Default {
                    n177 = Bundle By Name(cluster=T27 {"Procedure"=enum."Measure", "Parameter"=enum."XY-X", "Symmetric"=FALSE} ("input cluster"), "Procedure"=ProcedureState."Test") -> (w369:T27)
                  }
                  frame "Diffs and Distortion" {
                    n178 = Bundle By Name(cluster=T27 {"Procedure"=enum."Measure", "Parameter"=enum."XY-X", "Symmetric"=FALSE} ("input cluster"), "Procedure"=ProcedureState."Test") -> (w374:T27)
                  }
                  frame "Dwell Times" {
                    n179 = Bundle By Name(cluster=T27 {"Procedure"=enum."Measure", "Parameter"=enum."XY-X", "Symmetric"=FALSE} ("input cluster"), "Procedure"=ProcedureState."Test") -> (w378:T27)
                  }
                }
                n180 = call "Enqueue Message.vi"("Message Data"=w366, "Message"=w367, "Queue"=w364) -> ()  [unwired: 7 in, 2 out]
              }
            }
          }
        }
      }
      event "Testing Range (Norm)_min", "Testing Range (Norm)_max", "Auto Focus", "Search_max", "Search_min", "Calibration_max", "Calibration_min", "auto-set pockel", "Pockels Cell Value for pointing mode": Value Change {
        n181 = event-data() -> ()  [unwired: 1 in, 6 out]
      }
      event "Measure PSF": Value Change {
        n182 = event-data() -> ("NewVal"=w380:bool)  [unwired: 1 in]
        n183 = case shown="True" w380 {
          tunnel: w381 -> [_ w385]
          frame False {
          }
          frame True {
            n184 = Bundle By Name(cluster=T27 {"Procedure"=enum."Measure", "Parameter"=enum."XY-X", "Symmetric"=FALSE} ("input cluster"), "Procedure"=ProcedureState."Measure") -> (w384:T27)
            n185 = call "Enqueue Message.vi"("Message Data"=w384, "Message"="Measure PSF", "Queue"=w385) -> ()  [unwired: 7 in, 2 out]
          }
        }
      }
      event "Reload": Value Change {
        n186 = event-data() -> ("NewVal"=w390:bool)  [unwired: 1 in, 5 out]
        n187 = case shown="True" w390 {
          tunnel: "Current Calibration Parameters" -> [_ w409]
          tunnel: "Current Objective" -> [_ _]
          tunnel: [errorcluster {"status"=FALSE, "code"=0, "source"=""} ("error out") w393] -> w387
          frame False {
          }
          frame True {
            (unwired) T15."Image" ("Calibration Tab")
            n188 = call "fgv_calibration_config.vi"("Cal config ops"=T12."Load from file") -> ("error out"=w398:errorcluster, "File Path"=w394:path, "Config cluster OUT"=w395:T16)  [unwired: 8 in]
            n189 = control-ref of="Objectives"() -> (w397:refnum<vi>)
            n190 = Open/Create/Replace File(file path (use dialog)=w394) -> (refnum out=w404:refnum<file>, error out=w403:errorcluster)  [unwired: 5 in, 1 out]
            n191 = property on="Calibration.ini Path" class="Path"("Value"=w394) -> ()  [unwired: 2 in, 2 out]
            n192 = call "Update fgv objectives.vi"("error in (no error)"=w398, "Config cluster IN"=w395) -> ("Available Objectives"=w402:string[], "Current Objective"=w401:string)  [unwired: 7 in, 1 out]
            n193 = Read from Text File(file (use dialog)=w404, error in=w403) -> (refnum out=w405:refnum<file>, text=w396:string, error out=w406:errorcluster)  [unwired: 2 in, 1 out]
            n194 = call "Update Objective tree.vi"("Visible Items:Column Headers Visible"=TRUE, "error in (no error)"=w398, "Column Header Strings[]"=string[] ["Item", "Value"], "Config cluster IN"=w395, "TreeControl in"=w397) -> ("error out"=w393:errorcluster)  [unwired: 6 in]
            n195 = property on="Objective" class="CmbBox (strict)"("Strings[]"=w402, "Value"=w401) -> ()  [unwired: 2 in, 2 out]
            n196 = Close File(refnum=w405, error in=w406) -> ()  [unwired: 2 out]
            n197 = property on="Calibration.ini" class="Str"("Value"=w396) -> ()  [unwired: 2 in, 2 out]
            n198 = call "Update Objective calibration data.vi"("Config cluster OUT"=w395, "Current Calibration Parameters in"=w409) -> ("Current Calibration Parameters out"=w408:T8)  [unwired: 8 in, 1 out]
            n199 = property on="Calibration Tab" class="TabCtl (strict)"("Value"=T3."Live Image" ("Calibration Tab")) -> ()  [unwired: 2 in, 2 out]
            n200 = local write "Current Calibration Parameters"(w408) -> ()
          }
        }
      }
      event Value Change {
        n201 = event-data() -> ("OldVal"=w412:T8, "NewVal"=w410:T8)  [unwired: 1 in, 4 out]
        n202 = Not Equal?(x=w412, y=w410) -> (x != y?=w411:bool)
        n203 = case shown="True" w411 {
          tunnel: w410 -> [_ w413]
          frame False {
          }
          frame True {
            n204 = call "Update_Matlab_for_calib.vi"("Current Calibration Parameters"=w413) -> ()  [unwired: 10 in, 1 out]
          }
        }
      }
      event "Visible(Grid)", "Grid Lines": Value Change {
        n205 = event-data() -> ()  [unwired: 1 in, 1 out]
        n206 = case shown="True" "Visible(Grid)" {
          frame False {
            n207 = local read "Image"() -> (w416:T4)
            n208 = call "IMAQ Clear Overlay"("Image"=w416) -> ("Image Out"=w415:T4)  [unwired: 9 in, 1 out]
            n209 = local write "Image"(w415) -> ()
          }
          frame True {
            n210 = local read "Image"() -> (w423:T4)
            n211 = property class="IMAQImage"(reference=w423) -> (reference out=w420:T4, error out=w419:errorcluster, "ImageSize"=w422:cluster{"x":i32, "y":i32})  [unwired: 1 in]
            n212 = Unbundle By Name(w422) -> ("x"=w417:i32)
            n213 = Not Equal To 0?(x=w417) -> (x != 0?=w421:bool)
            n214 = case shown="True" w421 {
              tunnel: w420 -> [_ w427]
              tunnel: w419 -> [_ w426]
              tunnel: "Grid Lines" -> [_ w424]
              frame False {
              }
              frame True {
                n215 = call "Draw_Grid.vi"("error in (no error)"=w426, "Grid Lines"=w424, "Image In"=w427) -> ("Image Out"=w428:T4)  [unwired: 7 in, 1 out]
                n216 = local write "Visible(Grid)"(TRUE ("Visible(Grid)")) -> ()
                n217 = local write "Image"(w428) -> ()
              }
            }
          }
        }
      }
    }
  }
  "Stop_Ind" <- w23
  n218 = while {
    tunnel: w22 -> [w436]
    tunnel: w21 -> [w432]
    tunnel: w19 -> [_]
    tunnel: [w429] -> w4
    stop <- w429 stop-if-true
    n219 = call "Dequeue Message.vi"("Error In"=w432, "timeout in ms (-1)"=10, "Message Queue"=w436) -> ("Error Out"=w431:errorcluster, "Message Data"=w434:variant, "Message"=w435:string)  [unwired: 4 in, 2 out]
    n220 = case shown="\"Scaling\"" w435 {
      tunnel: w434 -> [_ _ _ w448 w457 w483 w487 w494 w504]
      tunnel: T27 {"Procedure"=enum."Measure", "Parameter"=enum."XY-X", "Symmetric"=FALSE} ("input cluster") -> [_ _ _ w447 w458 w482 w488 w493 w502]
      tunnel: w431 -> [_ w438 _ _ w455 _ w486 w495 _]
      tunnel: [w437 _ _ _ _ _ _ _ _] -> w429
      frame Default {
        n221 = local read "Stop_Ind"() -> (w437:bool)
      }
      frame "Exit" {
        n222 = disable-structure shown="Enabled" {
          disable-tunnel: [w442 w446] -> w439
          disable-tunnel: w438 -> [w440 w446]
          frame Disabled {
            n223 = global read "gl_Queues.vi" "UI queue name"() -> (w441:string)
            n224 = call "Obtain Message Queue.vi"("error in (no error)"=w440, "Queue name"=w441) -> ("error out"=w445:errorcluster, "Message Queue"=w444:refnum<queue>)  [unwired: 8 in]
            n225 = call "Enqueue Message.vi"("error in (no error)"=w445, "Message"="Unload subpanel", "Queue"=w444) -> ("error out"=w442:errorcluster)  [unwired: 7 in, 1 out]
          }
          frame Enabled {
          }
        }
        n226 = call <vilib>:"Simple Error Handler.vi"("error in (no error)"=w439) -> ()  [unwired: 4 in, 5 out]
      }
      frame "Initialize" {
      }
      frame "Measure PSF" {
        n227 = Variant To Data(type=w447, Variant=w448) -> (data=w449:T27)  [unwired: 1 in, 1 out]
        n228 = Unbundle By Name(w449) -> ()  [unwired: 1 out]
      }
      frame "Scaling" {
        n229 = Variant To Data(error in=w455, type=w458, Variant=w457) -> (data=w454:T27, error out=w456:errorcluster)
        n230 = local read "AOL Z values"() -> (w450:i32[])
        n231 = local read "Signal Channel"() -> (w452:enum16{"Red", "Green"})
        n232 = local read "Motor Z values"() -> (w451:i32[])
        n233 = Unbundle By Name(w454) -> ("Procedure"=w453:T2)
        n234 = disable-structure shown="Disabled" {
          disable-tunnel: w454 -> [w474 _]
          disable-tunnel: w456 -> [w473 _]
          frame Disabled {
            n235 = Unbundle By Name(w474) -> ("Parameter"=w469:T26)
            n236 = call "Calibrate_AOL XYZ.vi"("error in (no error)"=w473, "Stage Control"=w469) -> ("norm_to_um_scaling"=w470:dbl)  [unwired: 8 in, 1 out]
            n237 = case shown="\"Z\"" w469 {
              tunnel: [w477 w480] -> w472
              tunnel: T8 {"Sum X"=0.0, "Sum Y"=0.0, "Diff X"=0.0, "Diff Y"=0.0, "Distortion Correction"=0.0, "Z_norm to um_scaling"=0.0, "X_norm to um_scaling"=0.0, "Samples to Wait after Trigger"=0.0, "Slip Cycle"=0.0} ("Current Calibration Parameters") -> [w476 w479]
              tunnel: w470 -> [w475 w478]
              frame "Z" {
                n238 = Bundle By Name(cluster=w476, "Z_norm to um_scaling"=w475) -> (w477:T8)
              }
              frame "XY-X", Default {
                n239 = Bundle By Name(cluster=w479, "X_norm to um_scaling"=w478) -> (w480:T8)
              }
            }
            n240 = local write "Current Calibration Parameters"(w472) -> ()
          }
          frame Enabled {
          }
        }
        n241 = case shown="\"Calibrate\"" w453 {
          tunnel: w452 -> [_ w464 w468]
          tunnel: w451 -> [_ w463 _]
          tunnel: w450 -> [_ w462 _]
          frame "Measure", Default {
          }
          frame "Sequence" {
            w460 = T25 1 items=["Grayscale (U8)", "Grayscale (I16)", "Grayscale (SGL)", "Complex (CSG)", "RGB (U32)", "HSL (U32)", "RGB (U64)", "Grayscale (U16)"] ("Image Type")
            n242 = call "Get frame sequence.vi"("Signal Channel"=w464, "AOL Z values"=w462, "Motor Z values"=w463) -> ("Array"=w461:T4[])  [unwired: 7 in, 1 out]
            "Array" <- w461
            n243 = call "MaxZ from Image array.vi"("Image Type"=w460, "Array"=w461) -> ("Image 2"=w459:T4)  [unwired: 8 in, 1 out]
            n244 = local write "Image"(w459) -> ()
          }
          frame "Calibrate" {
            n245 = call "Get single frame.vi"("Signal Channel"=w468) -> ("Image"=w467:T4)  [unwired: 9 in, 1 out]
            n246 = call "IMAQ ImageToArray"("Image"=w467) -> ("Image Pixels (I16)"=w465:i16[][])  [unwired: 3 in, 4 out]
            "Image Pixels (I16)" <- w465
            "Intensity Graph" <- w465
            n247 = local write "Image"(w467) -> ()
            n248 = call-poly <vilib>:"Plot Helper.vi"("z matrix"=w465) -> ("3D Plot lvclass Array out"=→"3D Surface":refnum<class "3D Plot Datatype.lvclass">[])  [unwired: 5 in, 5 out]
          }
        }
      }
      frame "Sums" {
        n249 = Variant To Data(type=w482, Variant=w483) -> (data=w484:T27)  [unwired: 1 in, 1 out]
        n250 = Unbundle By Name(w484) -> ("Procedure"=w481:T2)
        "Procedure" <- w481
        n251 = case shown="\"Calibrate\"" w481 {
          frame "Test", Default {
          }
          frame "Calibrate" {
            n252 = local read "Signal Channel"() -> (w485:enum16{"Red", "Green"})
            n253 = call "Calibrate_Sums.vi"("Signal Channel"=w485) -> ()  [unwired: 8 in, 3 out]
          }
        }
      }
      frame "Diffs and Distortion" {
        n254 = Variant To Data(error in=w486, type=w488, Variant=w487) -> (data=w489:T27)  [unwired: 1 out]
        n255 = Unbundle By Name(w489) -> ()  [unwired: 1 out]
      }
      frame "Dwell Times" {
        n256 = Variant To Data(error in=w495, type=w493, Variant=w494) -> (data=w496:T27)  [unwired: 1 out]
        n257 = Unbundle By Name(w496) -> ("Procedure"=w492:T2)
        n258 = case shown="\"Test\"" w492 {
          tunnel: [w498 _] -> w491
          frame "Test" {
            w497 = u32 2 items=["Grayscale", "Binary", "Gradient", "Rainbow", "Temperature", "User Defined", "Binary 16 Bit", "Gradient 16 Bit", "Rainbow 16 Bit", "Temperature 16 Bit", "User Defined 16 Bit"] ("Palette:Palette Type")
            n259 = local read "Signal Channel"() -> (w501:enum16{"Red", "Green"})
            n260 = call "Test_Dwelltime.vi"("number of points"=4, "Signal Channel"=w501) -> ("error out"=w498:errorcluster, "MaxProj"=w500:T4)  [unwired: 8 in]
            n261 = property on="Image" class="ImageControl"(error in=w498, "Palette Type"=w497) -> ()  [unwired: 1 in, 2 out]
            n262 = local write "Image"(w500) -> ()
          }
          frame Default {
          }
        }
        n263 = call "Message_Update_Calib_frontpanel.vi"("error in (no error)"=w491, "Message"="Tested: Image is Updated") -> ()  [unwired: 9 in, 1 out]
      }
      frame "Magnification" {
        n264 = Variant To Data(type=w502, Variant=w504) -> (data=w503:T27)  [unwired: 1 in, 1 out]
        n265 = Unbundle By Name(w503) -> ()  [unwired: 1 out]
      }
    }
  }
  n266 = while {
    tunnel: w18 -> [w515]
    tunnel: w17 -> [w512]
    tunnel: [w510] -> w16
    stop <- w513 stop-if-true
    n267 = Dequeue Element(queue=w515, timeout in ms (-1)=250, error in (no error)=w512) -> (element=w514:T37, error out=w510:errorcluster)  [unwired: 2 out]
    n268 = case shown="\"Red\", Default" "Signal Channel" {
      tunnel: w514 -> [w517 w519]
      tunnel: [w516 w518] -> w508
      frame "Red", Default {
        n269 = Unbundle By Name(w517) -> ("Red channel"=w516:T4)
      }
      frame "Green" {
        n270 = Unbundle By Name(w519) -> ("Green channel"=w518:T4)
      }
    }
    n271 = local read "Grid Lines"() -> (w505:u32)
    n272 = Equal?(x=w508, y=T4 refnum) -> (x = y?=w506:bool)
    n273 = local read "Stop_Ind"() -> (w513:bool)
    n274 = case shown="False" w506 {
      tunnel: w508 -> [w522 _]
      tunnel: w505 -> [w520 _]
      frame False {
        n275 = call "Draw_Grid.vi"("Grid Lines"=w520, "Image In"=w522) -> ("Image Out"=→"Image":T4)  [unwired: 8 in, 1 out]
      }
      frame True {
      }
    }
  }
  n276 = flat-sequence {
    tunnel: w4 -> [_]
    frame #0 {
      # "Enables live imaging windows again after the loop has stopped as the user has exited"
      n277 = global read "gl_UI Ctrl Refs.vi" "UI ctrl refs"() -> (w525:T23)
      n278 = Unbundle By Name(w525) -> ("Live Imaging"=w524:refnum<vi>)
      n279 = property class="Bool (strict)"(reference=w524, "DisabledEnum"=T11."Enabled" ("Disabled")) -> ()  [unwired: 1 in, 2 out]
    }
  }
  n280 = call <vilib>:"Clear Errors.vi"("error in (no error)"=w16) -> ()  [unwired: 5 in, 2 out]
  n281 = control-ref of="Objectives"() -> (w1:refnum<vi>)
  n282 = global write "General Globals.vi" "Calibration Toolbox"(w20) -> ()
  n283 = call "Tree - Close reference.vi"("error in (no error)"=w2, "TreeControl in"=w1) -> ()  [unwired: 9 in, 1 out]
